vi "Extend Config.vi"(8 "error in":errorcluster, 10 "Additional Config":refnum<class "config-base.lvclass">, 11 "config-base in":refnum<class "config-base.lvclass">) -> (0 "error out":errorcluster, 3 "config-base out":refnum<class "config-base.lvclass">)   [LabVIEW 2022 SP3, in "hse-config.lvlib" / "config-base.lvclass"]
doc: "Adds or replaces own config keys and sections with the content from \"Additional Config\". \n\n____\nHAMPEL SOFTWARE ENGINEERING v3.8.0 (2023-12-18 14:41)"
uses:
  config-base.lvclass
  config-base.lvclass/config-base.ctl
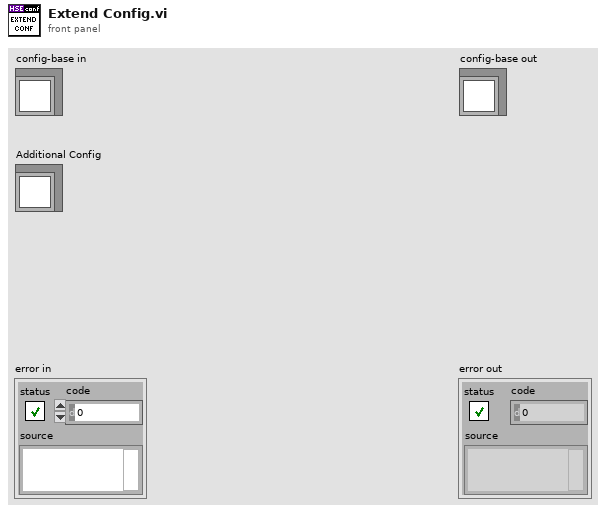
[diagram p1: front panel]
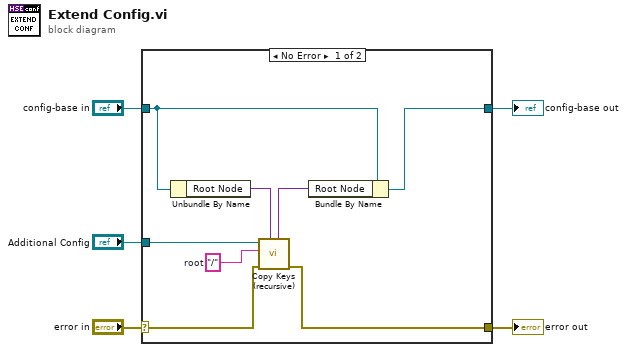
[diagram p0: block diagram]
diagram:
  n1 = case shown="No Error" "error in" {
    selector: "error in" -> [w11 w15]
    tunnel: [w8 w15] -> w4
    tunnel: [w7 w14] -> w2
    tunnel: "config-base in" -> [w13 w14]
    tunnel: "Additional Config" -> [w12 _]
    frame No Error {
      w10 = "/"  # root
      n2 = Unbundle By Name(w13) -> ("Root Node"=w9:variant)
      n3 = call "Copy Keys (recursive).vi"("Root Node in"=w9, "error in"=w11, "Section"=w10, "Additional Config"=w12) -> ("error out"=w8:errorcluster, "Root Node out"=w6:variant)  [unwired: 6 in]
      n4 = Bundle By Name(cluster=w13, "Root Node"=w6) -> (w7:refnum<class "config-base.lvclass">)
    }
    frame Error {
    }
  }
  "error out" <- w4
  "config-base out" <- w2
